vi "Arm calibration.vi"(7 "Cali. Power":i8=20, 8 "Down Power":i8=20, 9 "Rotation":i32=75, 11 "NXT/EV3":T1) -> (3 "NXT/EV3":T1)   [LabVIEW 2015]
uses:
  <vilib>/NXT/Block Support/NXT_OutputPort.ctl
  <vilib>/NXT/LegoClasses/BrickReference/BrickReference.lvclass
  <vilib>/NXT/Subs/LVHSConnector.ctl
  <vilib>/NXT/NXTIO Xnodes/NXTIOXNode/NXTIO.xnode
  <vilib>/NXT/NXTIO Xnodes/AddressXNode/NXTIOAddress.xnode
  <vilib>/NXT/NXTIO Xnodes/NXTIONodeSubVIs/NXTMoveMotors.vi
  <vilib>/NXT/Dual Mode Library/Waits/Wait_Touch.vi
  <vilib>/NXT/Block Support/NXT_InputPort.ctl
  <vilib>/NXT/NXTIO Xnodes/NXTIONodeSubVIs/NXTStopMotors.vi
  <vilib>/NXT/Dual Mode Library/Waits/Wait_Num.vi
  <vilib>/NXT/NXTIO Xnodes/NXTIONodeSubVIs/LEGOResetMotors.vi
  <vilib>/NXT/NXTIO Xnodes/NXTIONodeSubVIs/NXTMotorRunDistance.vi
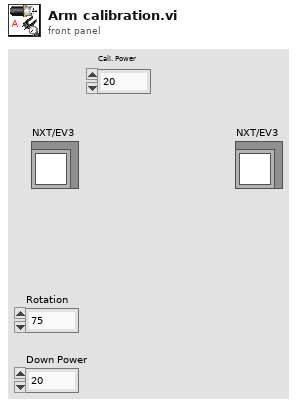
[diagram p1: front panel]
types:
  T1 = typedef "LVHSConnector.ctl" = refnum<class "BrickReference.lvclass">
  T2 = typedef "NXT_InputPort.ctl" = u32
  T3 = typedef "NXT_OutputPort.ctl" = u8
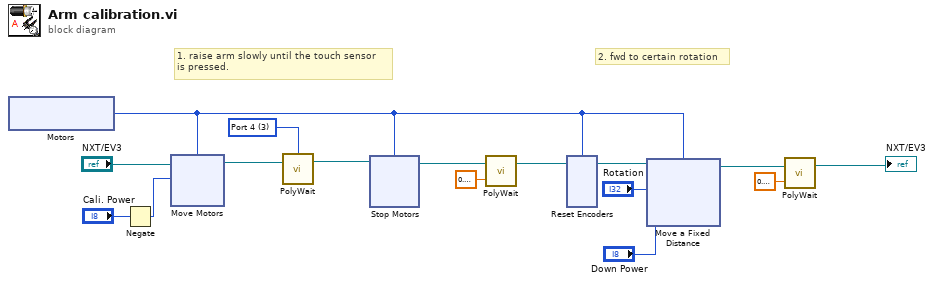
[diagram p0: block diagram]
diagram:
  w14 = T2 3 items=["Port 1", "Port 2", "Port 3", "Port 4"] ("Port (Port 1)")
  # "2. fwd to certain rotation"
  # "1. raise arm slowly until the touch sensor\nis pressed."
  n1 = xnode "Motors"() -> ("Motor"=w8:T3)
  n2 = Negate(x="Cali. Power") -> (-x=w1:i8)
  n3 = xnode "Move Motors"("Power/Speed 1"=w1, "Motors"=w8, "NXT/EV3"="NXT/EV3") -> ("NXT/EV3"=w15:T1)
  n4 = call-poly <vilib>:"PolyWait.vi"("NXT/EV3"=w15, "Port (Port 1)"=w14) -> ("NXT/EV3"=w13:T1)  [unwired: 2 in]
  n5 = xnode "Stop Motors"("Motors"=w8, "NXT/EV3"=w13) -> ("NXT/EV3"=w12:T1)
  n6 = call-poly <vilib>:"PolyWait.vi"("Time (1 sec)"=sgl 0.2, "NXT/EV3"=w12) -> ("NXT/EV3"=w10:T1)  [unwired: 2 in]
  n7 = xnode "Reset Encoders"("Motors"=w8, "NXT/EV3"=w10) -> ("NXT/EV3"=w9:T1)
  n8 = xnode "Move a Fixed Distance"("Speed 1"="Down Power", "Distance 1"="Rotation", "Motors"=w8, "NXT/EV3"=w9) -> ("NXT/EV3"=w3:T1)
  n9 = call-poly <vilib>:"PolyWait.vi"("Time (1 sec)"=sgl 0.2, "NXT/EV3"=w3) -> ("NXT/EV3"=→"NXT/EV3":T1)  [unwired: 2 in]
